vi "Fetch Current.vi"(0 "VISA resource name":refnum<visa-resource-name>, 11 "error in (no error)":errorcluster) -> (2 "Average Current":dbl, 3 "RMS Current":dbl, 4 "VISA resource name out":refnum<visa-resource-name>, 6 "High Current Level":dbl, 8 "Low Current Level":dbl, 13 "Maximum Current Level":dbl, 14 "Minimum Current Level":dbl, 15 "error out":errorcluster)   [LabVIEW 2021, in "Agilent N6900 N7900 Series.lvlib"]
doc: "Fetches current information from the instrument.\n\nNote:\nUse this VI only with other low-level VIs. The high-level VIs automatically incorporate this functionality. This VI does not check the instrument status."
uses:
  <instrlib>/Agilent N6900 N7900 Series/Agilent N6900 N7900 Series.lvlib
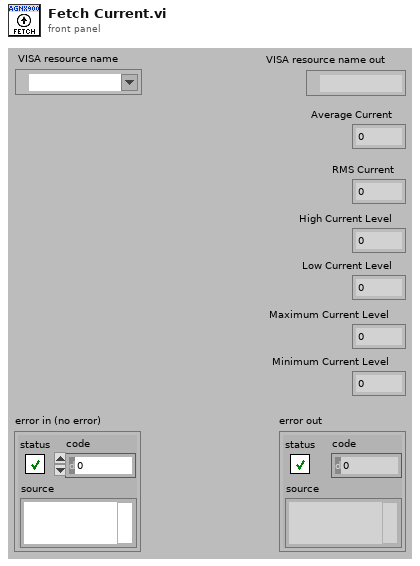
[diagram p1: front panel]
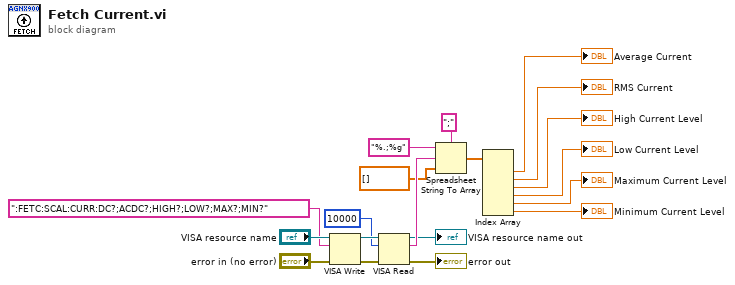
[diagram p0: block diagram]
diagram:
  n1 = VISA Write(VISA resource name="VISA resource name", write buffer=":FETC:SCAL:CURR:DC?;ACDC?;HIGH?;LOW?;MAX?;MIN?", error in (no error)="error in (no error)") -> (VISA resource name out=w15:refnum<visa-resource-name>, error out=w16:errorcluster)  [unwired: 1 out]
  n2 = VISA Read(VISA resource name=w15, byte count=u32 10000, error in (no error)=w16) -> (VISA resource name out=→"VISA resource name out":refnum<visa-resource-name>, read buffer=w13:string, error out=→"error out":errorcluster)  [unwired: 1 out]
  n3 = Spreadsheet String To Array(delimiter (Tab)=";", format string="%.;%g", spreadsheet string=w13, array type (2D Dbl)=dbl[] []) -> (array=w9:dbl[])
  n4 = Index Array(array=w9) -> (element #1=→"Average Current":dbl, element #2=→"RMS Current":dbl, element #3=→"High Current Level":dbl, element #4=→"Low Current Level":dbl, element #5=→"Maximum Current Level":dbl, element #6=→"Minimum Current Level":dbl)  [unwired: 6 in]
